vi "!CoMP-S Loop Delay.vi"(8 "error in (no error)":errorcluster, 11 "Delay (2000ms)":i32=2000) -> (0 "error out":errorcluster)   [LabVIEW 2014]
doc: "Use this template to build a VI to use as a subVI."
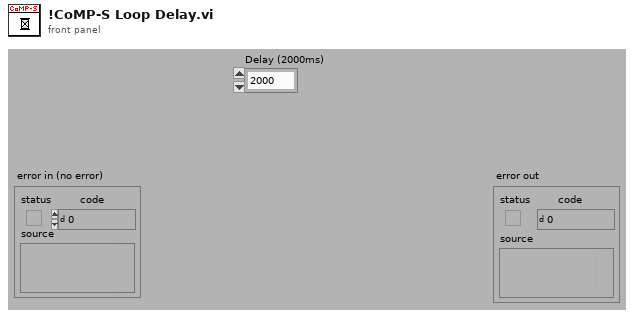
[diagram p1: front panel]
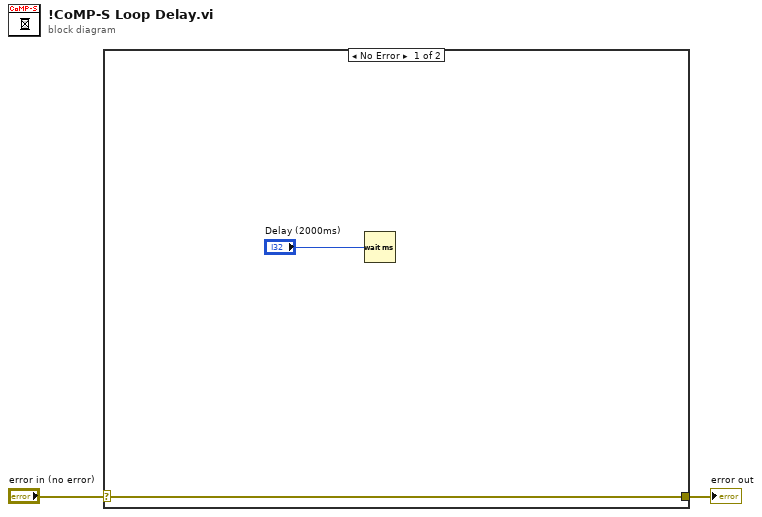
[diagram p0: block diagram]
diagram:
  n1 = case shown="No Error" "error in (no error)" {
    selector: "error in (no error)" -> [w3 w5]
    tunnel: [w3 w5] -> w1
    frame No Error {
      n2 = Wait (ms)(milliseconds to wait="Delay (2000ms)") -> ()  [unwired: 1 out]
    }
    frame Error {
    }
  }
  "error out" <- w1
